vi "Console_BufferSize.vi"(7 "Buffer Size":i32, 11 "Console Out in":string) -> (3 "Console Out out":string)   [LabVIEW 2022 SP3]
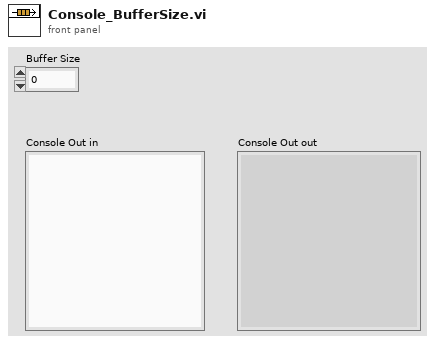
[diagram p1: front panel]
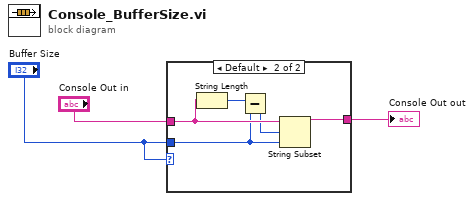
[diagram p0: block diagram]
diagram:
  n1 = case shown="Default" "Buffer Size" {
    tunnel: [w4 w9] -> w3
    tunnel: "Buffer Size" -> [_ w6]
    tunnel: "Console Out in" -> [w4 w7]
    frame -1 {
    }
    frame Default {
      n2 = String Length(string=w7) -> (length=w8:i32)
      n3 = Subtract(x=w8, y=w6) -> (x-y=w5:i32)
      n4 = String Subset(string=w7, offset (0)=w5, length (rest)=w6) -> (substring=w9:string)
    }
  }
  "Console Out out" <- w3
